vi "Set Limits.vi"(8 "error in (no error)":errorcluster, 11 "Stanford Research PS350 in":refnum<class "Stanford Research PS350.lvclass">) -> (0 "error out":errorcluster, 3 "Stanford Research PS350 out":refnum<class "Stanford Research PS350.lvclass">)   [LabVIEW 2011, in "Stanford Research PS350.lvclass"]
uses:
  Stanford Research PS350.lvclass
  Stanford Research PS350.lvclass/Stanford Research PS350.ctl
  3rd Party/Stanford Research PS300 Series/Stanford Research PS300 Series.lvlib
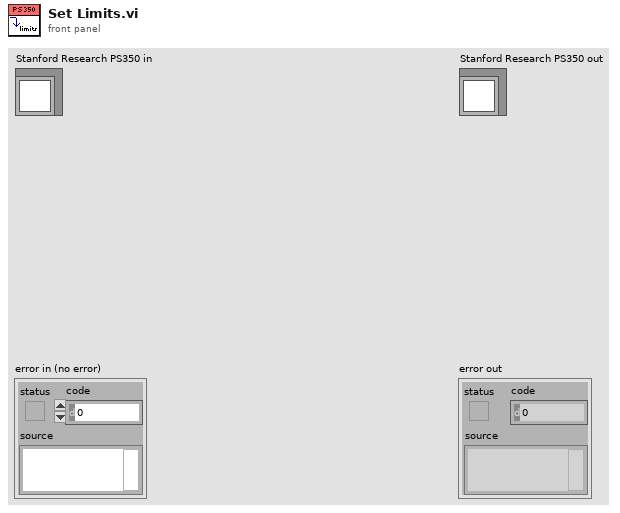
[diagram p1: front panel]
types:
  T1 = typedef "Power Supply.lvclass/Protection Limits.ctl" = cluster{"Voltage Limit":dbl, "Voltage Limit Units":T2, "Current Limit":dbl, "Current Limit Units":T3, "Voltage Trip/Cmpl":dbl, "Voltage Trip/Cmpl Units":T2, "Current Trip/Cmpl":dbl, "Current Trip/Cmpl Units":T3}
  T2 = typedef "Power Supply.lvclass/Voltage Units.ctl" = enum16{"volts", "millivolts", "microvolts"}
  T3 = typedef "Power Supply.lvclass/Current Units.ctl" = enum16{"amps", "milliamps", "microamps", "nanoamps"}
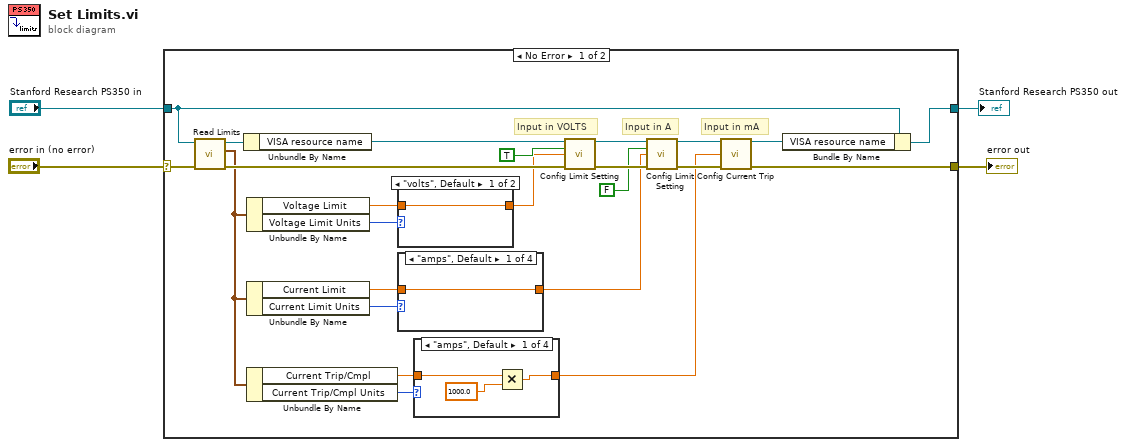
[diagram p0: block diagram]
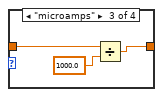
[diagram p3: hidden frame]
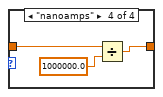
[diagram p4: hidden frame]
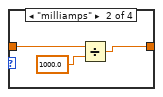
[diagram p5: hidden frame]
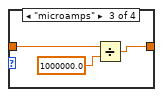
[diagram p6: hidden frame]
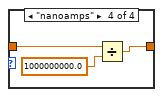
[diagram p7: hidden frame]
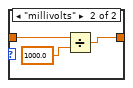
[diagram p8: hidden frame]
diagram:
  n1 = case shown="No Error" "error in (no error)" {
    selector: "error in (no error)" -> [w16 w54]
    tunnel: [w21 w54] -> w3
    tunnel: [w24 w53] -> w1
    tunnel: "Stanford Research PS350 in" -> [w18 w53]
    frame No Error {
      # "Input in mA"
      # "Input in A"
      # "Input in VOLTS"
      n2 = call-dynamic "Read Limits.vi"("error in (no error)"=w16, "Power Supply in"=w18) -> ("error out"=w15:errorcluster, "Protection Limits"=w8:T1, "Power Supply out"=w17:refnum<class "Stanford Research PS350.lvclass">)  [unwired: 7 in]
      n3 = Unbundle By Name(w17) -> ("VISA resource name"=w28:refnum<visa-resource-name>)
      n4 = Unbundle By Name(w8) -> ("Voltage Limit"=w13:dbl, "Voltage Limit Units"=w14:T2)
      n5 = Unbundle By Name(w8) -> ("Current Limit"=w10:dbl, "Current Limit Units"=w11:T3)
      n6 = Unbundle By Name(w8) -> ("Current Trip/Cmpl"=w7:dbl, "Current Trip/Cmpl Units"=w6:T3)
      n7 = case shown="\"volts\", Default" w14 {
        tunnel: w13 -> [w49 w51]
        tunnel: [w49 w52] -> w12
        frame "volts", Default {
        }
        frame "millivolts" {
          n8 = Divide(x=w51, y=1000.0) -> (x/y=w52:dbl)
        }
      }
      n9 = case shown="\"amps\", Default" w11 {
        tunnel: w10 -> [w39 w41 w45 w47]
        tunnel: [w39 w42 w43 w46] -> w9
        frame "amps", Default {
        }
        frame "milliamps" {
          n10 = Divide(x=w41, y=1000.0) -> (x/y=w42:dbl)
        }
        frame "microamps" {
          n11 = Divide(x=w45, y=1000000.0) -> (x/y=w43:dbl)
        }
        frame "nanoamps" {
          n12 = Divide(x=w47, y=1000000000.0) -> (x/y=w46:dbl)
        }
      }
      n13 = case shown="\"amps\", Default" w6 {
        tunnel: w7 -> [w31 w32 w35 w37]
        tunnel: [w30 w32 w33 w36] -> w5
        frame "amps", Default {
          n14 = Multiply(x=w31, y=1000.0) -> (x*y=w30:dbl)
        }
        frame "milliamps" {
        }
        frame "microamps" {
          n15 = Divide(x=w35, y=1000.0) -> (x/y=w33:dbl)
        }
        frame "nanoamps" {
          n16 = Divide(x=w37, y=1000000.0) -> (x/y=w36:dbl)
        }
      }
      n17 = call "Config Limit Setting.vi"("VISA resource name"=w28, "Source Setting (T:Voltage)"=TRUE, "High Limit (1.00E+3)"=w12, "error in (no error)"=w15) -> ("VISA resource name out"=w27:refnum<visa-resource-name>, "error out"=w23:errorcluster)  [unwired: 10 in]
      n18 = call "Config Limit Setting.vi"("VISA resource name"=w27, "Source Setting (T:Voltage)"=FALSE, "High Limit (1.00E+3)"=w9, "error in (no error)"=w23) -> ("VISA resource name out"=w26:refnum<visa-resource-name>, "error out"=w22:errorcluster)  [unwired: 10 in]
      n19 = call "Config Current Trip.vi"("VISA resource name"=w26, "Trip Value (5.25 mA)"=w5, "error in (no error)"=w22) -> ("VISA resource name out"=w25:refnum<visa-resource-name>, "error out"=w21:errorcluster)  [unwired: 11 in]
      n20 = Bundle By Name(cluster=w18, "VISA resource name"=w25) -> (w24:refnum<class "Stanford Research PS350.lvclass">)
    }
    frame Error {
    }
  }
  "error out" <- w3
  "Stanford Research PS350 out" <- w1
